vi "ArmExecute.vi"(8 "error in (no error)":errorcluster) -> (0 "error out":errorcluster)   [LabVIEW 2023]
doc: "Arm Execute for 2024 robot"
uses:
  ArmGetSetpointEnum.ctl
  <vilib>/Rock Robotics/WPI/ThirdParty/JAS_Junk/TrajLib/VI/BoolCmd_Recv_Internal.vi
  <vilib>/Rock Robotics/WPI/ThirdParty/JAS_Junk/TrajLib/VI/BoolCmd_ObtainQueue.vi
  Climb/ClimbGlobal.vi
  ArmNetworkingGlobal.vi
  ArmGlobal.vi
  <vilib>/Rock Robotics/WPI/ThirdParty/JAS_Junk/TrajLib/Trajectory_Library.lvlib
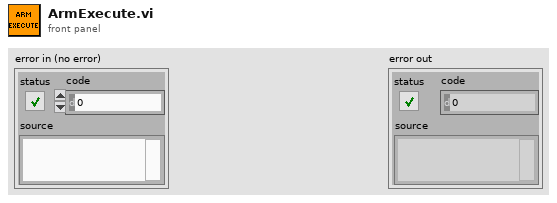
[diagram p1: front panel]
types:
  T1 = typedef "WPI_MotorControlDeviceRef.ctl" = cluster{"DeviceStatus":errorcluster, "Type":T2, "PWM":cluster{"PWM Channel":T3, "DeadBand":T4}, "CAN":cluster{"Device Number":u8, "SetOutput VI Ref":variant, "GetOutput VI Ref":variant, "Enable VI Ref":variant, "Disable VI Ref":variant, "Data":variant}, "Invert":bool, "DIO PWM":cluster{"PWM \"Enable\" Channel":T3, "DIOChannel":T5, "PWM Rate":dbl}}
  T2 = typedef "WPI_MotorControlType.ctl" = enum16{"PWM", "CAN", "DIO PWM"}
  T3 = typedef "FPGA_DIOPWMChannel.ctl" = enum8{"PWM 0", "PWM 1", "PWM 2", "PWM 3", "PWM 4", "PWM 5", "PWM 6", "PWM 7", "PWM 8", "PWM 9", "PWM MXP 0", "PWM MXP 1", "PWM MXP 2", "PWM MXP 3", "PWM MXP 4", "PWM MXP 5", "PWM MXP 6", "PWM MXP 7", "PWM MXP 8", "PWM MXP 9", "Invalid"}
  T4 = typedef "WPI_PWMDeadband.ctl" = cluster{"Name":string, "maxPositivePwm":i32, "minPositivePwm":i32, "centerPwm":i32, "maxNegativePwm":i32, "minNegativePwm":i32, "angularRange":u16}
  T5 = typedef "FPGA_DIOChannel.ctl" = enum8{"DIO 0", "DIO 1", "DIO 2", "DIO 3", "DIO 4", "DIO 5", "DIO 6", "DIO 7", "DIO 8", "DIO 9", "DIO MXP 0", "DIO MXP 1", "DIO MXP 2", "DIO MXP 3", "DIO MXP 4", "DIO MXP 5", "DIO MXP 6", "DIO MXP 7", "DIO MXP 8", "DIO MXP 9", "DIO MXP 10", "DIO MXP 11", "DIO MXP 12", "DIO MXP 13", "DIO MXP 14", "DIO MXP 15", "SPI Port CS1", "SPI Port CS2", "SPI Port CS3", "SPI Port MISO", "SPI Port MOSI", "Invalid"}
  T6 = typedef "WPI_SwitchDevRef.ctl" = cluster{"DevStatus":errorcluster, "DIO Channel":T5, "CntIndex":T7, "Normally Closed":bool}
  T7 = typedef "FPGA_CounterCtrSystemIndex.ctl" = enum8{"Ctr 0", "Ctr 1", "Ctr 2", "Ctr 3", "Ctr 4", "Ctr 5", "Ctr 6", "Ctr 7", "Invalid"}
  T8 = typedef "ArmGetSetpointEnum.ctl" = enum16{"ArmFloorPickup", "ArmAmpDeposit", "ArmSpeakerShoot", "ArmStartPosition", "ArmRestPosition", "ArmSourceIntake", "ArmAwayShoot"}
  T9 = typedef "Trajectory_Library.lvlib/PosCtrl_Tuning_Type.ctl" = cluster{"Slope":dbl, "Offset":dbl, "Error Deadband":dbl, "At Reference Count":i32, "Negate Output":bool, "Max Allowd Position":dbl, "Min Allowd Position":dbl}
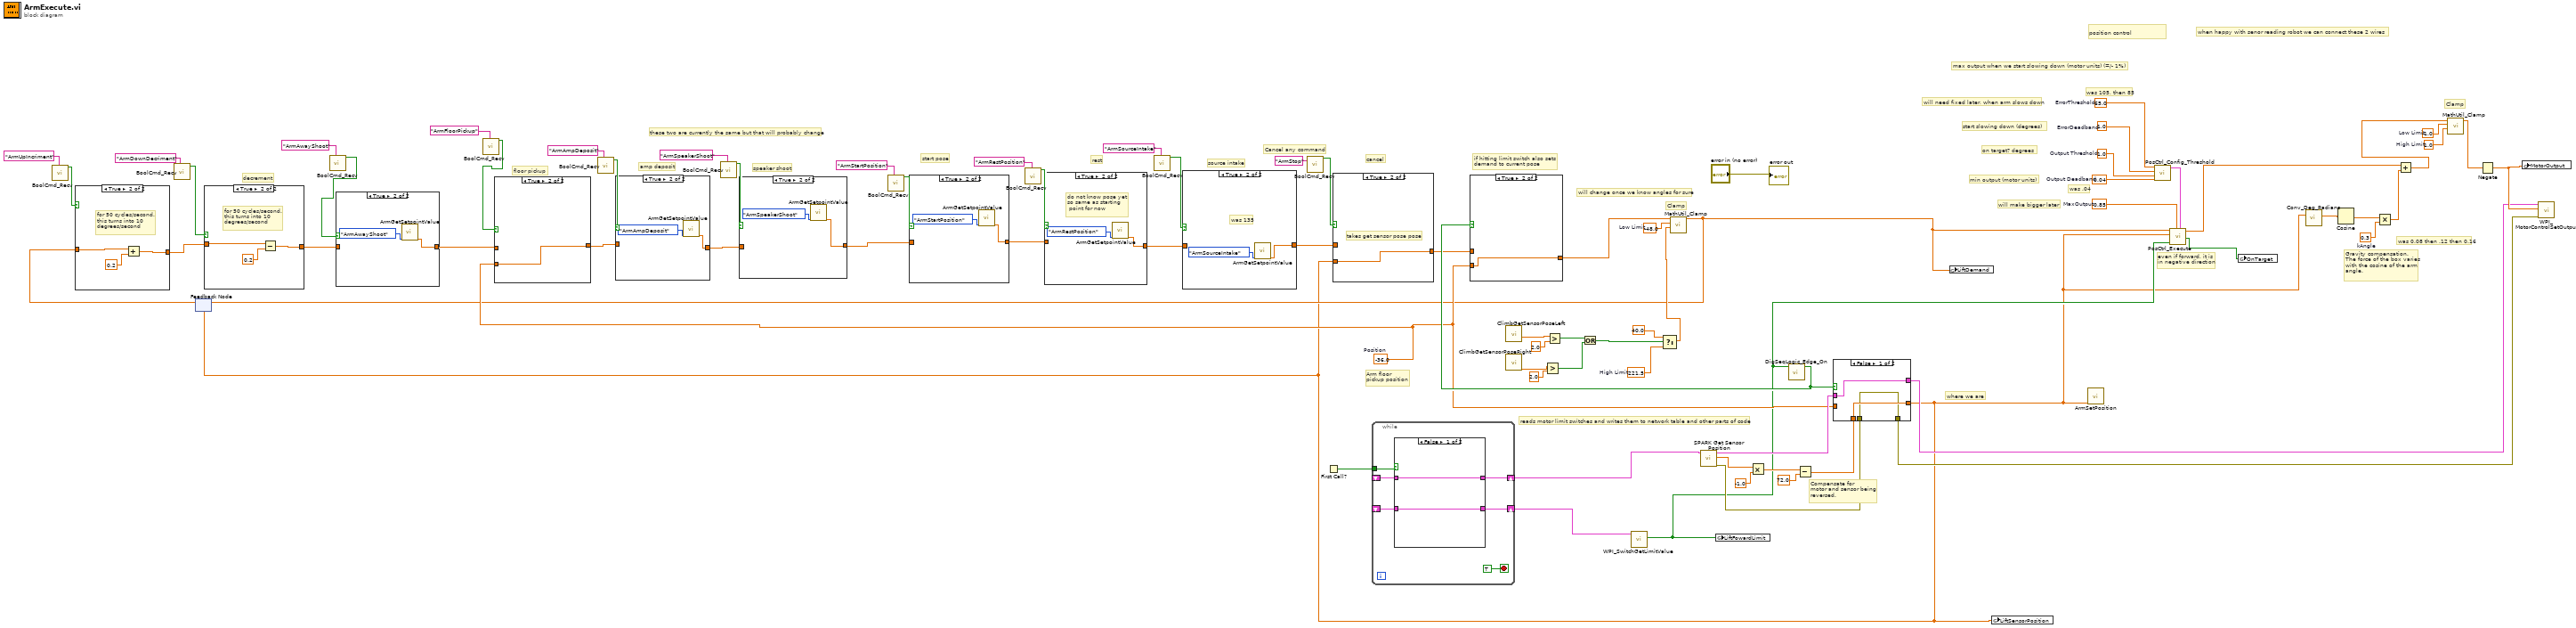
[diagram p0: block diagram]
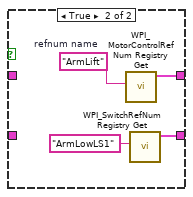
[diagram p2: hidden frame]
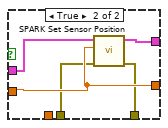
[diagram p14: hidden frame]
diagram:
  w5 = 1.0  # High Limit
  w4 = -1.0  # Low Limit
  w18 = 221.5  # High Limit
  w31 = -36.0  # Position
  w43 = 0.3  # kAngle
  w69 = -48.0  # Low Limit
  w78 = 0.85  # MaxOutput
  w76 = 65.0  # ErrorThreshold
  w75 = 1.0  # ErrorDeadband
  w74 = 1.0  # Output Threshold
  w73 = 0.04  # Output Deadband
  # "Clamp"
  # "was 105, then 85"
  # "was .04"
  # "was 0.08 then .12 then 0.16"
  # "Arm floor\npickup position"
  # "Gravity compensation.\nThe force of the box varies\nwith the cosine of the arm\nangle."
  # "Compensate for\nmotor and sensor being\nreversed."
  # "even if forward, it is \nin negative direction"
  # "if hitting limit switch also sets \ndemand to current pose"
  # "these two are currently the same but that will probably change"
  # "Cancel any command"
  # "source intake"
  # "will change once we know angles for sure"
  # "cancel"
  # "rest"
  # "start pose"
  # "speaker shoot"
  # "Clamp"
  # "amp deposit"
  # "floor pickup"
  # "decrement"
  # "when happy with senor reading robot we can connect these 2 wires"
  # "min output (motor units)"
  # "max output when we start slowing down (motor units) (=/- 1%)"
  # "on target? degrees"
  # "start slowing down (degrees)"
  # "will make bigger later"
  # "where we are"
  # "position control"
  # "will need fixed later, when arm slows down"
  # "reads motor limit switches and writes them to network table and other parts of code"
  n1 = call <vilib>:"BoolCmd_Recv.vi"("Command Name"="ArmUpIncriment") -> ("New Request"=w62:bool)  [unwired: 9 in, 1 out]
  n2 = call <vilib>:"BoolCmd_Recv.vi"("Command Name"="ArmDownDecriment") -> ("New Request"=w60:bool)  [unwired: 9 in, 1 out]
  n3 = call <vilib>:"BoolCmd_Recv.vi"("Command Name"="ArmAwayShoot") -> ("New Request"=w26:bool)  [unwired: 9 in, 1 out]
  n4 = call <vilib>:"BoolCmd_Recv.vi"("Command Name"="ArmFloorPickup") -> ("New Request"=w27:bool)  [unwired: 9 in, 1 out]
  n5 = call <vilib>:"BoolCmd_Recv.vi"("Command Name"="ArmAmpDeposit") -> ("New Request"=w57:bool)  [unwired: 9 in, 1 out]
  n6 = call <vilib>:"BoolCmd_Recv.vi"("Command Name"="ArmSpeakerShoot") -> ("New Request"=w55:bool)  [unwired: 9 in, 1 out]
  n7 = call <vilib>:"BoolCmd_Recv.vi"("Command Name"="ArmStartPosition") -> ("New Request"=w53:bool)  [unwired: 9 in, 1 out]
  n8 = call <vilib>:"BoolCmd_Recv.vi"("Command Name"="ArmRestPosition") -> ("New Request"=w51:bool)  [unwired: 9 in, 1 out]
  n9 = call <vilib>:"BoolCmd_Recv.vi"("Command Name"="ArmSourceIntake") -> ("New Request"=w49:bool)  [unwired: 9 in, 1 out]
  n10 = call <vilib>:"BoolCmd_Recv.vi"("Command Name"="ArmStop") -> ("New Request"=w47:bool)  [unwired: 9 in, 1 out]
  n11 = First Call?() -> (First Call?: T/F=w15:bool)
  n12 = while {
    tunnel: w15 -> [w83]
    shift-right: [w84] -> w6
    shift-left: _ -> [w81]
    shift-right: [w80] -> w10
    shift-left: _ -> [w79]
    stop <- TRUE stop-if-true
    n13 = case shown="False" w83 {
      tunnel: [w86 w90] -> w84
      tunnel: w81 -> [w86 _]
      tunnel: [w85 w87] -> w80
      tunnel: w79 -> [w85 _]
      frame False {
      }
      frame True {
        w89 = "ArmLift"  # refnum name
        n14 = call <vilib>:"WPI_MotorControlRefNum Registry Get.vi"("refnum name"=w89) -> ("MotorControlDevRef"=w90:T1)  [unwired: 9 in, 1 out]
        n15 = call <vilib>:"WPI_SwitchRefNum Registry Get.vi"("refnum name"="ArmLowLS1") -> ("SwitchDevRef"=w87:T6)  [unwired: 9 in, 1 out]
      }
    }
  }
  n16 = call "ClimbGetSensorPoseLeft.vi"() -> ("ClimbGetSensorPoseLeft"=w25:dbl)  [unwired: 11 in]
  n17 = call "ClimbGetSensorPoseRight.vi"() -> ("ClimbGetSensorPoseRight"=w22:dbl)  [unwired: 11 in]
  n18 = Greater?(x=w22, y=2.0) -> (0:w20:bool)
  n19 = Greater?(x=w25, y=2.0) -> (0:w21:bool)
  n20 = Or(x=w21, y=w20) -> (x .or. y?=w19:bool)
  n21 = call <vilib>:"WPI_SwitchGetLimitValue.vi"("SwitchDevRef"=w10) -> ("Switch Pressed"=w9:bool)  [unwired: 8 in, 2 out]
  n22 = Select(t=40.0, s=w19, f=w18) -> (s? t:f=w16:dbl)
  n23 = call <vilib>:"SPARK Get Sensor Position.vi"("MotorControlDevRef in"=w6) -> ("error out"=w14:errorcluster, "Sensor Position"=w39:dbl, "MotorControlDevRef out"=w40:T1)  [unwired: 7 in, 1 out]
  n24 = global write "ArmNetworkingGlobal.vi" "LiftFowardLimit"(w9) -> ()
  n25 = Multiply(x=w39, y=-1.0) -> (x*y=w37:dbl)
  n26 = call <vilib>:"DigSeqLogic_Edge_On.vi"("Input"=w9) -> ("On Edge"=w34:bool)  [unwired: 10 in]
  n27 = Subtract(x=w37, y=72.0) -> (x-y=w35:dbl)
  n28 = case shown="False" w34 {
    tunnel: [w92 w98] -> w8
    tunnel: [w93 w96] -> w1
    tunnel: w35 -> [w93 _]
    tunnel: w40 -> [w92 w97]
    tunnel: w31 -> [_ w96]
    tunnel: w14 -> [w91 w95]
    tunnel: [w91 w94] -> w7
    frame False {
    }
    frame True {
      n29 = call <vilib>:"SPARK Set Sensor Position.vi"("error in"=w95, "Position"=w96, "MotorControlDeviceRef"=w97) -> ("error out"=w94:errorcluster, "MotorControlDeviceRef"=w98:T1)  [unwired: 7 in]
    }
  }
  n30 = feedback #1(w1) -> (w72:dbl)
  n31 = case shown="True" w62 {
    tunnel: w72 -> [w99 w102]
    tunnel: [w99 w100] -> w71
    frame False {
    }
    frame True {
      # "for 50 cycles/second.\nthis turns into 10 \ndegrees/second"
      n32 = Add(x=w102, y=0.2) -> (x+y=w100:dbl)
    }
  }
  n33 = case shown="True" w60 {
    tunnel: w71 -> [w103 w105]
    tunnel: [w103 w104] -> w30
    frame False {
    }
    frame True {
      # "for 50 cycles/second.\nthis turns into 10 \ndegrees/second"
      n34 = Subtract(x=w105, y=0.2) -> (x-y=w104:dbl)
    }
  }
  n35 = case shown="True" w26 {
    tunnel: w30 -> [w107 _]
    tunnel: [w107 w108] -> w29
    frame False {
    }
    frame True {
      n36 = call "ArmGetSetpointValue.vi"("ArmSetpoints"=ArmGetSetpointEnum."ArmAwayShoot") -> ("Setpoint"=w108:dbl)  [unwired: 10 in]
    }
  }
  n37 = case shown="True" w27 {
    tunnel: w29 -> [w110 _]
    tunnel: [w110 w111] -> w70
    tunnel: w31 -> [_ w111]
    frame False {
    }
    frame True {
    }
  }
  n38 = case shown="True" w57 {
    tunnel: w70 -> [w112 _]
    tunnel: [w112 w113] -> w68
    frame False {
    }
    frame True {
      n39 = call "ArmGetSetpointValue.vi"("ArmSetpoints"=ArmGetSetpointEnum."ArmAmpDeposit") -> ("Setpoint"=w113:dbl)  [unwired: 10 in]
    }
  }
  n40 = case shown="True" w55 {
    tunnel: w68 -> [w115 _]
    tunnel: [w115 w116] -> w67
    frame False {
    }
    frame True {
      n41 = call "ArmGetSetpointValue.vi"("ArmSetpoints"=ArmGetSetpointEnum."ArmSpeakerShoot") -> ("Setpoint"=w116:dbl)  [unwired: 10 in]
    }
  }
  n42 = case shown="True" w53 {
    tunnel: w67 -> [w118 _]
    tunnel: [w118 w119] -> w66
    frame False {
    }
    frame True {
      n43 = call "ArmGetSetpointValue.vi"("ArmSetpoints"=ArmGetSetpointEnum."ArmStartPosition") -> ("Setpoint"=w119:dbl)  [unwired: 10 in]
    }
  }
  n44 = case shown="True" w51 {
    tunnel: w66 -> [w121 _]
    tunnel: [w121 w122] -> w65
    frame False {
    }
    frame True {
      # "do not know pose yet \nso same as starting\n point for now"
      n45 = call "ArmGetSetpointValue.vi"("ArmSetpoints"=ArmGetSetpointEnum."ArmRestPosition") -> ("Setpoint"=w122:dbl)  [unwired: 10 in]
    }
  }
  n46 = case shown="True" w49 {
    tunnel: w65 -> [w124 _]
    tunnel: [w124 w125] -> w64
    frame False {
    }
    frame True {
      # "was 135"
      n47 = call "ArmGetSetpointValue.vi"("ArmSetpoints"=ArmGetSetpointEnum."ArmSourceIntake") -> ("Setpoint"=w125:dbl)  [unwired: 10 in]
    }
  }
  n48 = case shown="True" w47 {
    tunnel: w64 -> [w127 _]
    tunnel: [w127 w128] -> w32
    tunnel: w1 -> [_ w128]
    frame False {
    }
    frame True {
      # "takes get sensor pose pose"
    }
  }
  n49 = case shown="True" w34 {
    tunnel: w31 -> [_ w130]
    tunnel: [w129 w130] -> w33
    tunnel: w32 -> [w129 _]
    frame False {
    }
    frame True {
    }
  }
  n50 = call <vilib>:"MathUtil_Clamp.vi"("High Limit"=w16, "Low Limit"=w69, "Value"=w33) -> ("Result"=w11:dbl)  [unwired: 8 in]
  n51 = feedback-in #1(w11) -> ()
  n52 = global write "ArmNetworkingGlobal.vi" "LiftDemand"(w11) -> ()
  n53 = global write "ArmNetworkingGlobal.vi" "LiftSensorPosition"(w1) -> ()
  n54 = call "ArmSetPosition.vi"("ArmPos"=w1) -> ()  [unwired: 11 in]
  n55 = call <vilib>:"PosCtrl_Config_Threshold.vi"("Output Deadband"=w73, "Output Threshold"=w74, "ErrorDeadband"=w75, "ErrorThreshold"=w76) -> ("PosCtrl_Config_Params"=w77:T9)  [unwired: 7 in]
  n56 = call <vilib>:"PosCtrl_Execute.vi"("PosCtrl_Config_Params"=w77, "MaxOutput"=w78, "Rev Limit Switch"=w9, "CurrentPosition"=w1, "TargetPosition"=w11) -> ("OnTarget"=w12:bool, "Output"=w45:dbl)  [unwired: 4 in, 1 out]
  n57 = global write "ArmNetworkingGlobal.vi" "OnTarget"(w12) -> ()
  n58 = call <vilib>:"Conv_Deg_Radians.vi"("Degress"=w1) -> ("Radians"=w41:dbl)  [unwired: 10 in]
  n59 = Cosine(x=w41) -> (cos(x)=w42:dbl)
  n60 = Multiply(x=w42, y=w43) -> (x*y=w44:dbl)
  n61 = Add(x=w45, y=w44) -> (x+y=w3:dbl)
  n62 = call <vilib>:"MathUtil_Clamp.vi"("High Limit"=w5, "Low Limit"=w4, "Value"=w3) -> ("Result"=w2:dbl)  [unwired: 8 in]
  n63 = Negate(x=w2) -> (-x=w13:dbl)
  n64 = global write "ArmNetworkingGlobal.vi" "MotorOutput"(w13) -> ()
  n65 = call <vilib>:"WPI_MotorControlSetOutput.vi"("error in (no error)"=w7, "Output"=w13, "MotorControlDevRef"=w8) -> ()  [unwired: 6 in, 3 out]
  "error out" <- "error in (no error)"
